vi "ControllerUtil_GetModulusError.vi"(8 "Maximum_Input":dbl, 9 "Minimum_Input":dbl, 10 "Measurerment(PV)":dbl, 11 "Reference(SP)":dbl) -> (3 "Error":dbl)   [LabVIEW 2019, in "Trajectory_Library.lvlib"]
doc: "Returns modulus of error where error is the difference between the reference and a measurement.\nThis is used for continuous systems, for example rotational systems.\n\nInputs:\n - Reference (SP) -- Reference input of a controller\n - Measurement (PV) -- The current measurement.\n - MinimumInput -- The minimum value expected from the input.\n - MaximumInput -- The maximum value expected from the input.\n\nOutputs:\n - Error -- Error value of a continuous system."
uses:
  Trajectory_Library.lvlib
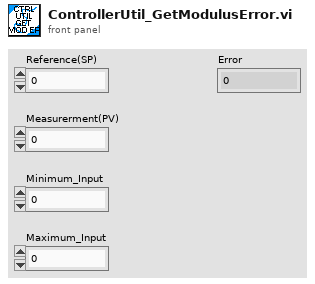
[diagram p1: front panel]
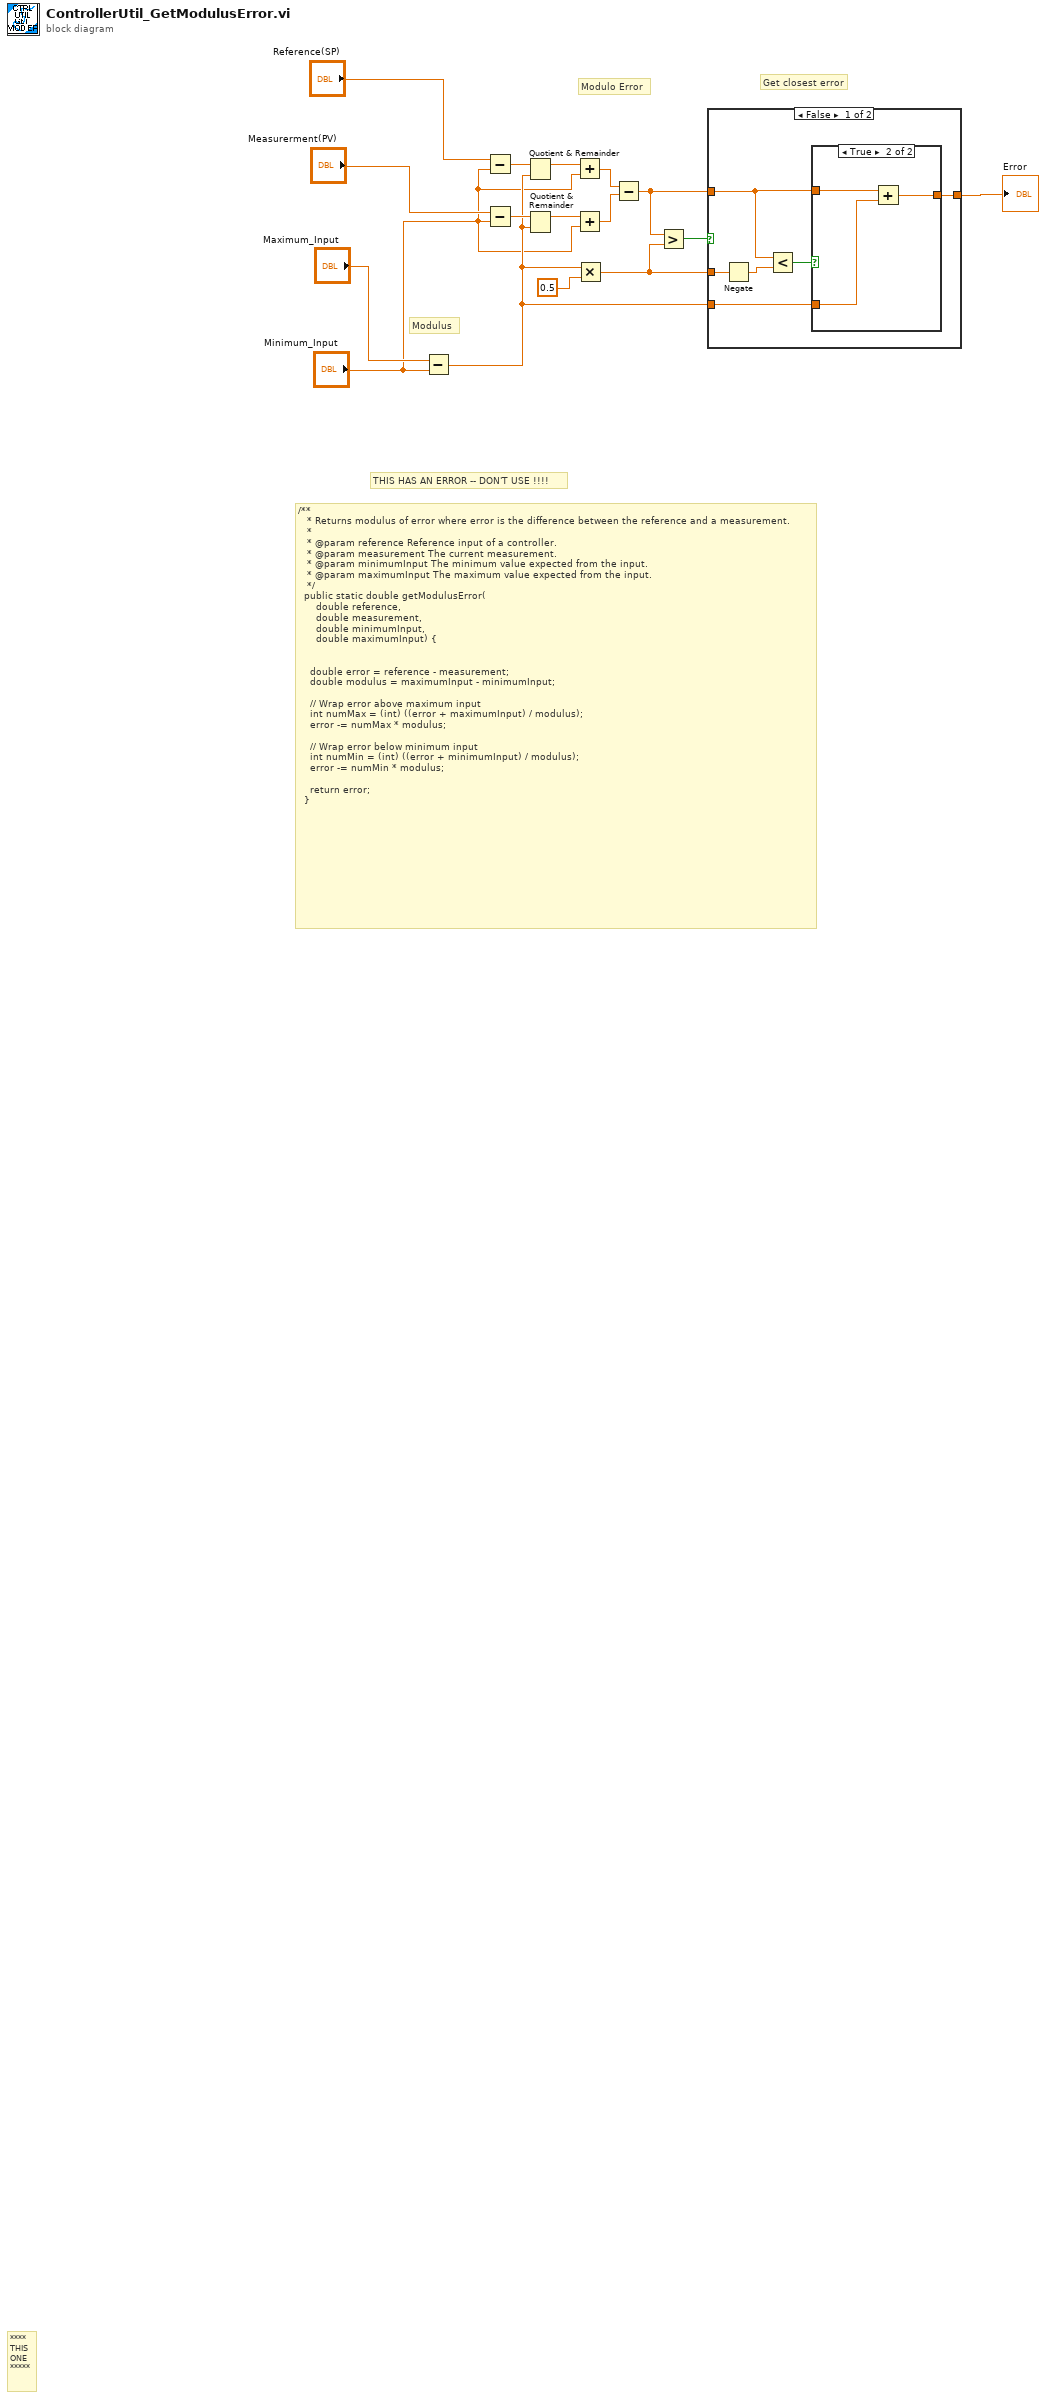
[diagram p0: block diagram]
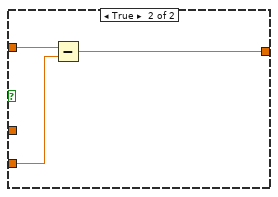
[diagram p3: hidden frame]
diagram:
  # "Modulus"
  # "Get closest error"
  # "Modulo Error"
  # "THIS HAS AN ERROR -- DON'T USE !!!!"
  # "/**\n   * Returns modulus of error where error is the difference between the reference and a measurement.\n   *\n   * @param reference Reference input of a controller.\n   * @param measurement The current measurement.\n   * @param minimumInput The minimum value expected from the input.\n   * @param maximumInput The maximum value expected from the input.\n   */\n  public static double getModulusError(\n      double reference, \n      double measurement, \n      double minimumInput, \n      double maximumInput) {\n\n\n    double error = reference - measurement;\n    double modulus = maximumInput - minimumInput;\n\n    // Wrap error above maximum input\n    int numMax = (int) ((error + maximumInput) / modulus);\n    error -= numMax * modulus;\n\n    // Wrap error below minimum input\n    int numMin = (int) ((error + minimumInput) / modulus);\n    error -= numMin * modulus;\n\n    return error;\n  }"
  # "****\nTHIS\nONE\n*****"
  n1 = Subtract(x="Maximum_Input", y="Minimum_Input") -> (x-y=w2:dbl)
  n2 = Subtract(x="Reference(SP)", y="Minimum_Input") -> (x-y=w11:dbl)
  n3 = Subtract(x="Measurerment(PV)", y="Minimum_Input") -> (x-y=w12:dbl)
  n4 = Quotient & Remainder(x=w11, y=w2) -> (x-y*floor(x/y)=w16:dbl)  [unwired: 1 out]
  n5 = Quotient & Remainder(x=w12, y=w2) -> (x-y*floor(x/y)=w15:dbl)  [unwired: 1 out]
  n6 = Add(x=w16, y="Minimum_Input") -> (x+y=w14:dbl)
  n7 = Add(x=w15, y="Minimum_Input") -> (x+y=w13:dbl)
  n8 = Multiply(x=w2, y=0.5) -> (x*y=w7:dbl)
  n9 = Subtract(x=w14, y=w13) -> (x-y=w8:dbl)
  n10 = Greater?(x=w8, y=w7) -> (0:w9:bool)
  n11 = case shown="False" w9 {
    tunnel: w2 -> [w19 w29]
    tunnel: w8 -> [w17 w28]
    tunnel: [w18 w27] -> w6
    tunnel: w7 -> [w22 _]
    frame False {
      n12 = Negate(x=w22) -> (-x=w21:dbl)
      n13 = Less?(x=w17, y=w21) -> (x < y?=w20:bool)
      n14 = case shown="True" w20 {
        tunnel: w19 -> [_ w24]
        tunnel: [w23 w26] -> w18
        tunnel: w17 -> [w23 w25]
        frame False {
        }
        frame True {
          n15 = Add(x=w25, y=w24) -> (x+y=w26:dbl)
        }
      }
    }
    frame True {
      n16 = Subtract(x=w28, y=w29) -> (x-y=w27:dbl)
    }
  }
  "Error" <- w6
